vi "GetBDObjects.vi"(8 "error in":errorcluster, 11 "VI Interpreter in":refnum<class "VI Interpreter.lvclass">) -> (0 "error out":errorcluster, 3 "VI Interpreter out":refnum<class "VI Interpreter.lvclass">)   [LabVIEW 2014, in "Raspberry Pi Compatible Compiler for LabVIEW.lvlib" / "VI Interpreter.lvclass"]
uses:
  VI Interpreter.lvclass
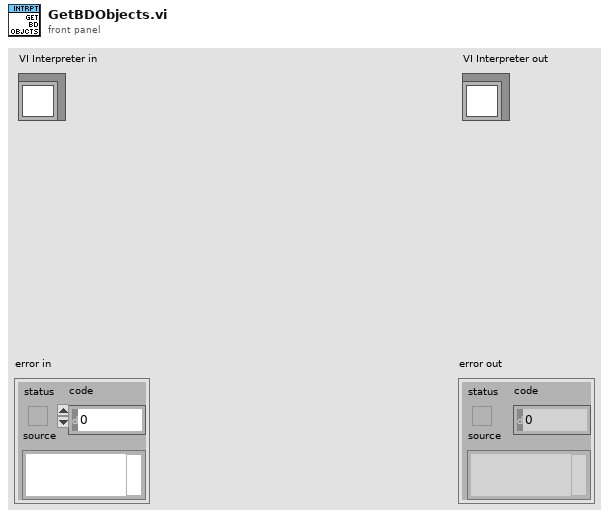
[diagram p1: front panel]
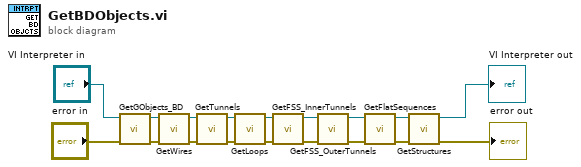
[diagram p0: block diagram]
diagram:
  n1 = call "GetGObjects_BD.vi"("error in"="error in", "VI Interpreter in"="VI Interpreter in") -> ("error out"=w18:errorcluster, "VI Interpreter out"=w17:refnum<class "VI Interpreter.lvclass">)  [unwired: 8 in]
  n2 = call "GetWires.vi"("error in"=w18, "VI Interpreter in"=w17) -> ("error out"=w16:errorcluster, "VI Interpreter out"=w15:refnum<class "VI Interpreter.lvclass">)  [unwired: 6 in]
  n3 = call "GetTunnels.vi"("error in"=w16, "VI Interpreter in"=w15) -> ("error out"=w11:errorcluster, "VI Interpreter out"=w12:refnum<class "VI Interpreter.lvclass">)  [unwired: 6 in]
  n4 = call "GetLoops.vi"("error in"=w11, "VI Interpreter in"=w12) -> ("error out"=w5:errorcluster, "VI Interpreter out"=w6:refnum<class "VI Interpreter.lvclass">)  [unwired: 6 in]
  n5 = call "GetFSS_InnerTunnels.vi"("error in"=w5, "VI Interpreter in"=w6) -> ("error out"=w3:errorcluster, "VI Interpreter out"=w4:refnum<class "VI Interpreter.lvclass">)  [unwired: 6 in]
  n6 = call "GetFSS_OuterTunnels.vi"("error in"=w3, "VI Interpreter in"=w4) -> ("error out"=w1:errorcluster, "VI Interpreter out"=w2:refnum<class "VI Interpreter.lvclass">)  [unwired: 6 in]
  n7 = call "GetFlatSequences.vi"("error in"=w1, "VI Interpreter in"=w2) -> ("error out"=w9:errorcluster, "VI Interpreter out"=w10:refnum<class "VI Interpreter.lvclass">)  [unwired: 6 in]
  n8 = call "GetStructures.vi"("error in"=w9, "VI Interpreter in"=w10) -> ("error out"=→"error out":errorcluster, "VI Interpreter out"=→"VI Interpreter out":refnum<class "VI Interpreter.lvclass">)  [unwired: 6 in]
